vi "SetTermination.vi"(7 "TerminationData":T1, 8 "Error In":errorcluster, 11 "GenAlg_data":T2={"BasicCondfig"={"parameters_range"=[], "Initial elements"=0}, "elements"=[], "CostFunction"=refnum, "GenerationData"={"ElementsCreated"=0}, "SelectionData"={"ElementsSelected"=0}, "SimulatedAnnealingData"={"AnnealingFactor"=0.0, "Active"=FALSE}, "CostFunctionData"=variant(refnum<vi> refnum), "MultiEval_data"={"Active"=FALSE, "MultiEvalFunction"=refnum}, "TerminationData"={"MaxGen"={"Generations"=0, "Active"=FALSE}, "CostFunctionTol"={"Tol"=0.0, "Active"=FALSE}, "GensEstab"={"Generations"=0, "Active"=FALSE}}}) -> (0 "Error Out":errorcluster, 3 "GenAlg_data-out":T2={"BasicCondfig"={"parameters_range"=[], "Initial elements"=0}, "elements"=[], "CostFunction"=refnum, "GenerationData"={"ElementsCreated"=0}, "SelectionData"={"ElementsSelected"=0}, "SimulatedAnnealingData"={"AnnealingFactor"=0.0, "Active"=FALSE}, "CostFunctionData"=variant(refnum<vi> refnum), "MultiEval_data"={"Active"=FALSE, "MultiEvalFunction"=refnum}, "TerminationData"={"MaxGen"={"Generations"=0, "Active"=FALSE}, "CostFunctionTol"={"Tol"=0.0, "Active"=FALSE}, "GensEstab"={"Generations"=0, "Active"=FALSE}}})   [LabVIEW 2016]
uses:
  TypeDefs/GenAlg_data.ctl
  TypeDefs/basic_config.ctl
  TypeDefs/element.ctl
  TypeDefs/geration_data.ctl
  TypeDefs/selection_data.ctl
  TypeDefs/SimulatedAnnealing_data.ctl
  TypeDefs/multi_eval_data.ctl
  TypeDefs/termination_data.ctl
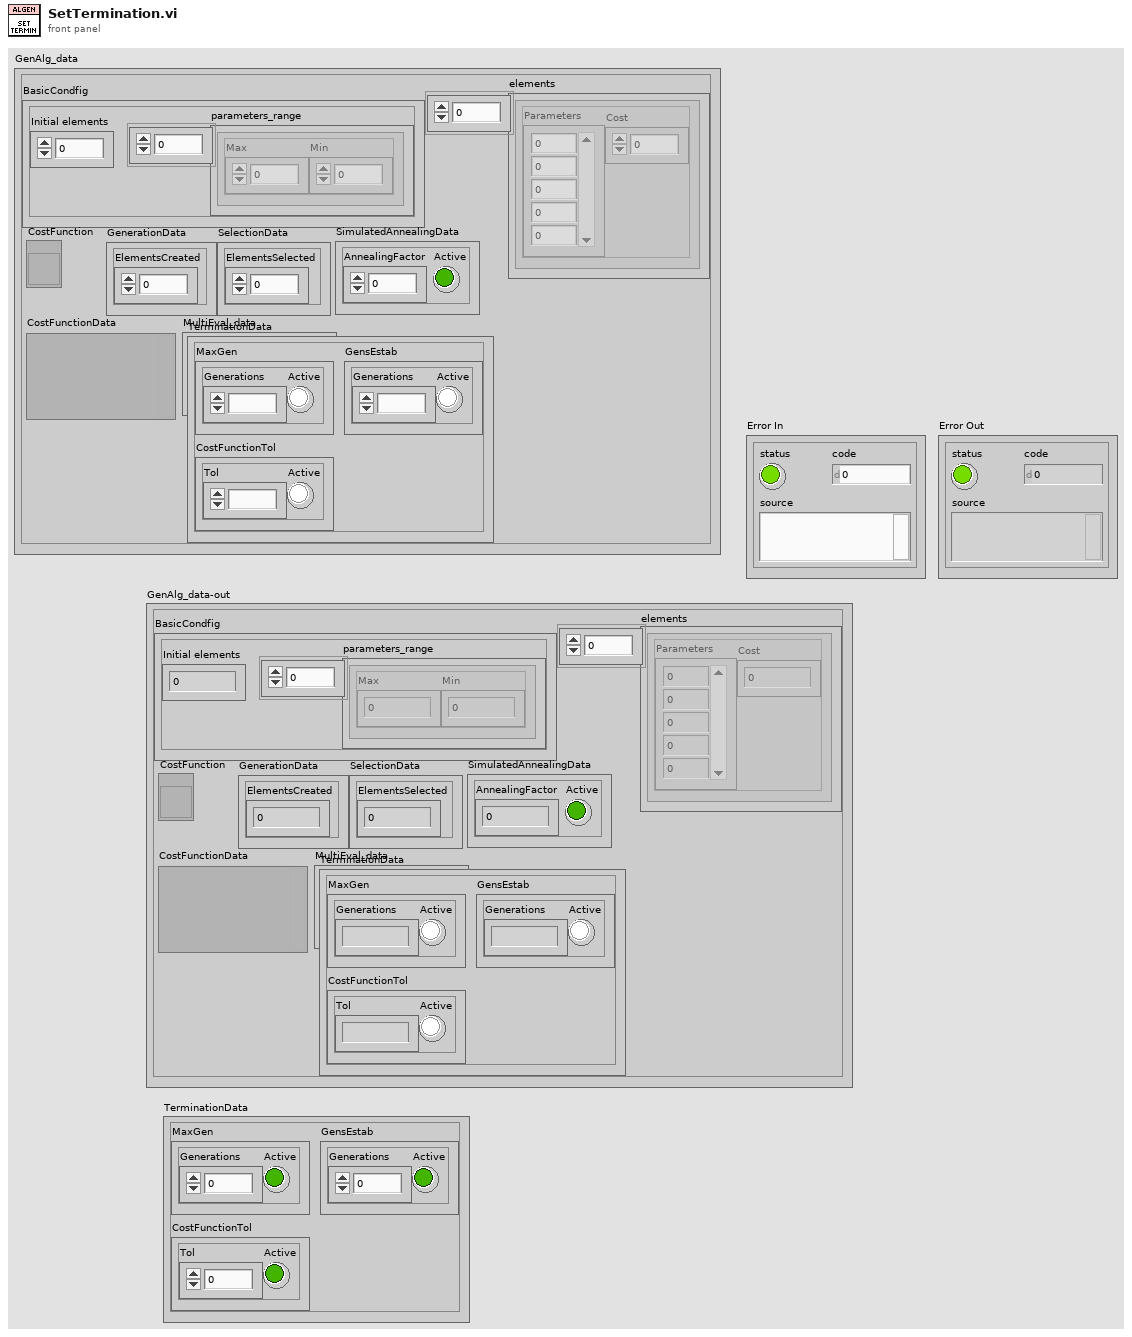
[diagram p1: front panel]
types:
  T1 = typedef "termination_data.ctl" = cluster{"MaxGen":cluster{"Generations":i32, "Active":bool}, "CostFunctionTol":cluster{"Tol":dbl, "Active":bool}, "GensEstab":cluster{"Generations":i32, "Active":bool}}
  T2 = typedef "GenAlg_data.ctl" = cluster{"BasicCondfig":T3, "elements":T4[], "CostFunction":refnum<vi>, "GenerationData":T5, "SelectionData":T6, "SimulatedAnnealingData":T7, "CostFunctionData":variant, "MultiEval_data":T8, "TerminationData":T1}
  T3 = typedef "basic_config.ctl" = cluster{"parameters_range":cluster{"Max":dbl, "Min":dbl}[], "Initial elements":i32}
  T4 = typedef "element.ctl" = cluster{"Parameters":dbl[], "Cost":dbl}
  T5 = typedef "geration_data.ctl" = cluster{"ElementsCreated":i32}
  T6 = typedef "selection_data.ctl" = cluster{"ElementsSelected":i32}
  T7 = typedef "SimulatedAnnealing_data.ctl" = cluster{"AnnealingFactor":dbl, "Active":bool}
  T8 = typedef "multi_eval_data.ctl" = cluster{"Active":bool, "MultiEvalFunction":refnum<vi>}
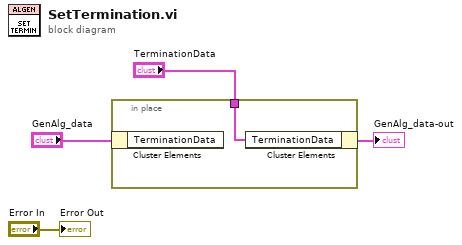
[diagram p0: block diagram]
diagram:
  n1 = in-place {
    in-place-border: "TerminationData" -> [w5]
    n2 = in-place-cluster #1("GenAlg_data") -> ()  [unwired: 1 out]
    n3 = in-place-cluster #1("TerminationData"=w5) -> (→"GenAlg_data-out":T2)
  }
  "Error Out" <- "Error In"
